vi "Read Booster Valve Gain Settings.vi"(8 "error in (no error)":errorcluster, 11 "Boot Loader in":refnum<class "Boot Loader.lvclass">) -> (0 "error out":errorcluster, 2 "ForceActuatorBoosterValveGainSettings":T1, 3 "Boot Loader out":refnum<class "Boot Loader.lvclass">)   [LabVIEW 2016]
uses:
  Boot Loader.lvclass
  Typedefs/ForceActuatorBoosterValveGainSettings.ctl
  Settings/Settings.lvclass
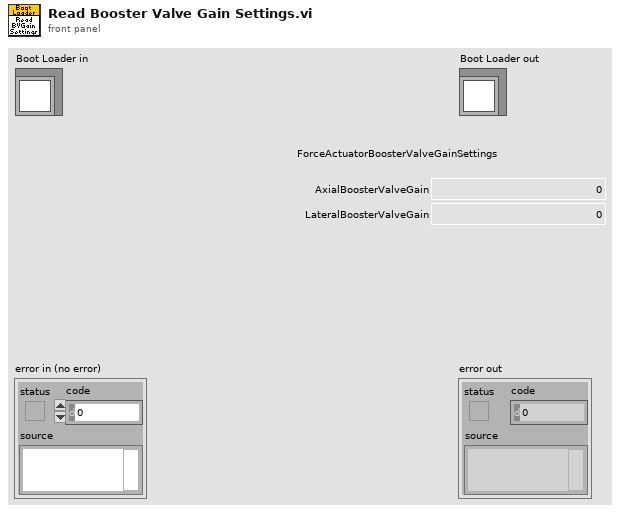
[diagram p1: front panel]
types:
  T1 = typedef "ForceActuatorBoosterValveGainSettings.ctl" = cluster{"AxialBoosterValveGain":sgl, "LateralBoosterValveGain":sgl}
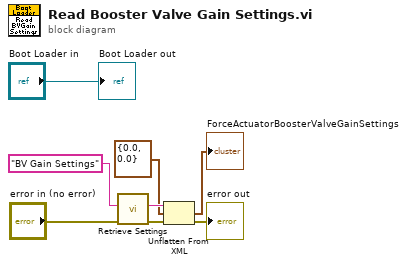
[diagram p0: block diagram]
diagram:
  n1 = call "Retrieve Settings.vi"("error in (no error)"="error in (no error)", "configName"="BV Gain Settings") -> ("error out"=w4:errorcluster, "xmlConfig"=w7:string)  [unwired: 7 in, 1 out]
  n2 = Unflatten From XML(xml string=w7, type=T1 {"AxialBoosterValveGain"=0.0, "LateralBoosterValveGain"=0.0} ("ForceActuatorBoosterValveGainSettings"), error in (no error)=w4) -> (value=→"ForceActuatorBoosterValveGainSettings":T1, error out=→"error out":errorcluster)
  "Boot Loader out" <- "Boot Loader in"
